vi "CreateWO-CompileDatatoSend.vi"(7 "Work Order":string, 8 "error in":errorcluster, 11 "ERP-CreateWorkOrder in":refnum<class "ERP-CreateWorkOrder.lvclass">) -> (0 "error out":errorcluster, 2 "Output JSON to DB":string, 3 "ERP-CreateWorkOrder out":refnum<class "ERP-CreateWorkOrder.lvclass">)   [LabVIEW 2013, in "ERP-CreateWorkOrder.lvclass"]
uses:
  ERP-CreateWorkOrder.lvclass
  ERP-CreateWorkOrder.lvclass/ERP-CreateWorkOrder.ctl
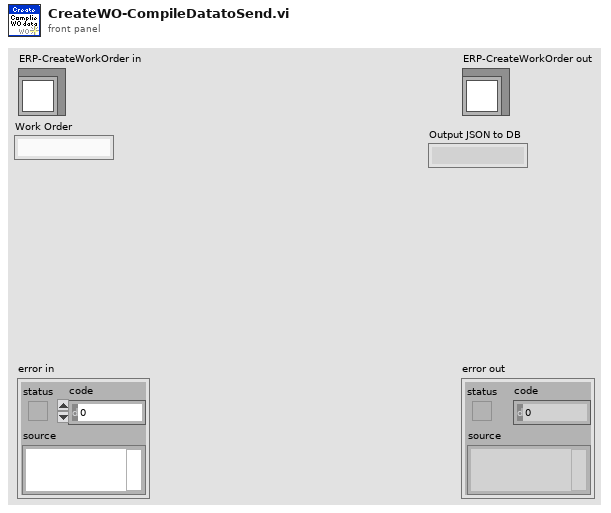
[diagram p1: front panel]
types:
  T1 = cluster{"Work Order":string, "Customer*":string, "Converted Start Date (String)":string, "Converted Due Date (String)":string, "Type Part Number*":string, "Part Number Description":string, "Quantity To Make":string, "Note - Special Instructions":string, "Assigned?":string, "Date Created":string, "Sales Order*":string, "Date Closed":string, "Status of Work Order":string, "Manufactured":string, "Inspected":string, "Approved":string, "Total Time to Manufacture":string, "Total Time to Inspect":string, "Path For PDF Special Instructions":string, "Reason For Closure":string, "RMA":string, "Manufacture User Notes":string, "Inspector User Notes":string, "Pull Inventory Note":string, "Stock Inventory Note":string}
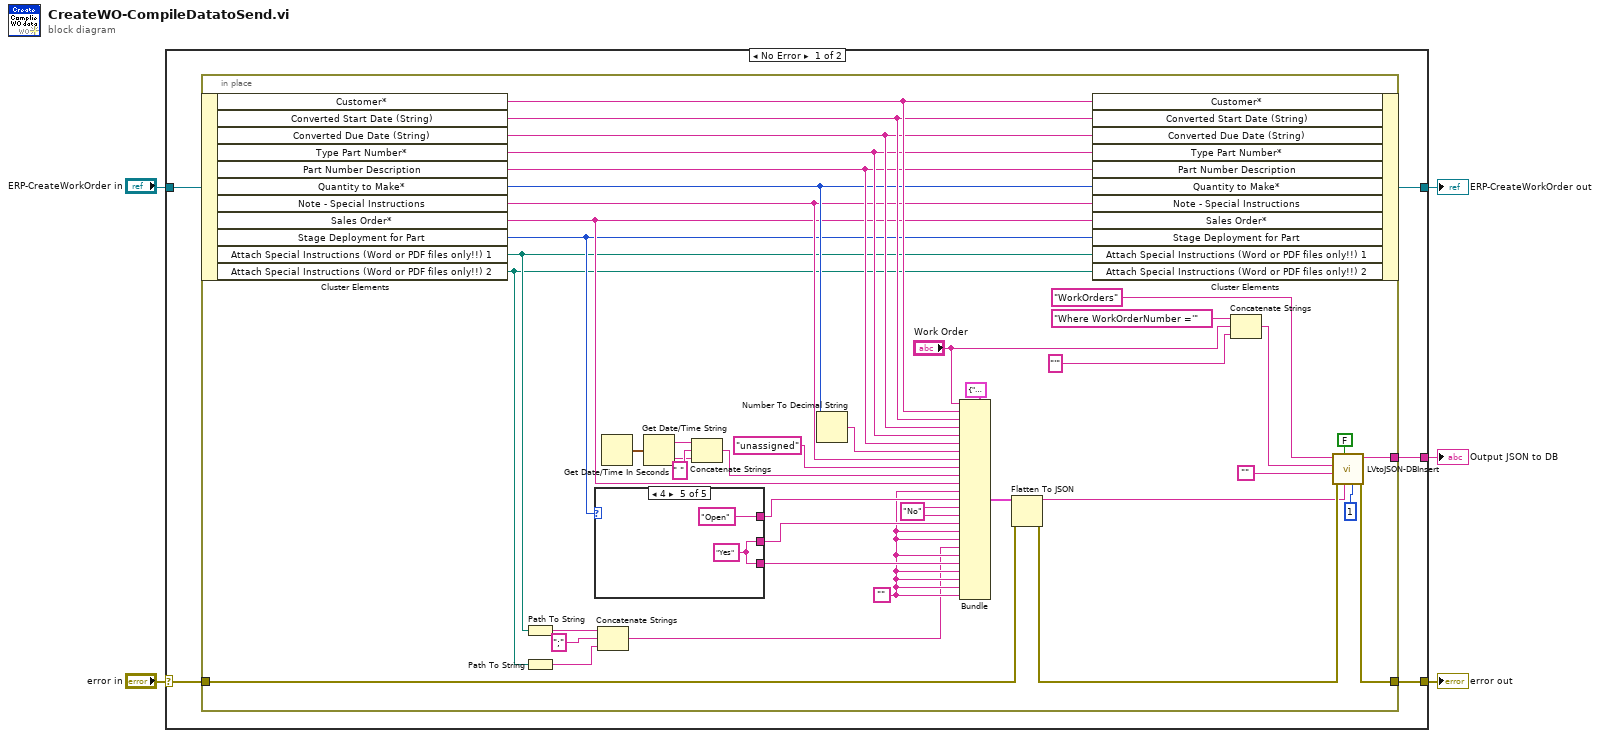
[diagram p0: block diagram]
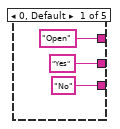
[diagram p2: hidden frame]
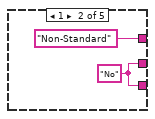
[diagram p3: hidden frame]
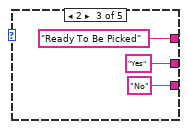
[diagram p4: hidden frame]
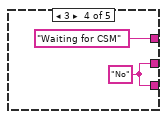
[diagram p5: hidden frame]
diagram:
  n1 = case shown="No Error" "error in" {
    selector: "error in" -> [w8 w66]
    tunnel: [w7 w66] -> w4
    tunnel: [w9 w65] -> w2
    tunnel: "ERP-CreateWorkOrder in" -> [w10 w65]
    tunnel: [w6 _] -> w1
    frame No Error {
      n2 = in-place {
        in-place-border: w8 -> [w17]
        in-place-border: [w30] -> w7
        in-place-border: [w29] -> w6
        w44 = "No" ("string")
        w25 = ""
        n3 = in-place-cluster #1(w10) -> ("Customer*"=w41:string, "Converted Start Date (String)"=w40:string, "Converted Due Date (String)"=w39:string, "Type Part Number*"=w38:string, "Part Number Description"=w37:string, "Quantity to Make*"=w36:i32, "Note - Special Instructions"=w35:string, "Sales Order*"=w34:string, "Stage Deployment for Part"=w33:u16, "Attach Special Instructions (Word or PDF files only!!) 1"=w24:path, "Attach Special Instructions (Word or PDF files only!!) 2"=w23:path)
        n4 = Path To String(path=w24) -> (string=w22:string)
        n5 = Path To String(path=w23) -> (string=w20:string)
        n6 = case shown="4" w33 {
          tunnel: ["Open" ("Status of Work Order") "Non-Standard" ("Status of Work Order") "Ready To Be Picked" ("Status of Work Order") "Waiting for CSM" ("Status of Work Order") "Open" ("Status of Work Order")] -> w45
          tunnel: ["Yes" ("Assigned?") w56 "Yes" ("Assigned?") w61 w63] -> w43
          tunnel: ["No" ("Assigned?") w56 "No" ("Assigned?") w61 w63] -> w42
          frame 0, Default {
          }
          frame 1 {
            w56 = "No" ("Assigned?")
          }
          frame 2 {
          }
          frame 3 {
            w61 = "No" ("Assigned?")
          }
          frame 4 {
            w63 = "Yes" ("Assigned?")
          }
        }
        n7 = Concatenate Strings(w22, ";" ("string"), w20) -> (w19:string)
        n8 = Get Date/Time In Seconds() -> (seconds since 1Jan1904=w50:timestamp)
        n9 = Get Date/Time String(seconds (now)=w50) -> (date string=w49:string, time string=w47:string)  [unwired: 2 in]
        n10 = Concatenate Strings(w49, " " ("string"), w47) -> (w46:string)
        n11 = Number To Decimal String(number=w36) -> (decimal integer string=w52:string)  [unwired: 1 in]
        n12 = Bundle(cluster=T1 {"Work Order"="", "Customer*"="", "Converted Start Date (String)"="", "Converted Due Date (String)"="", "Type Part Number*"="", "Part Number Description"="", "Quantity To Make"="", "Note - Special Instructions"="", "Assigned?"="", "Date Created"="", "Sales Order*"="", "Date Closed"="", "Status of Work Order"="", "Manufactured"="", "Inspected"="", "Approved"="", "Total Time to Manufacture"="", "Total Time to Inspect"="", "Path For PDF Special Instructions"="", "Reason For Closure"="", "RMA"="", "Manufacture User Notes"="", "Inspector User Notes"="", "Pull Inventory Note"="", "Stock Inventory Note"=""}, "Work Order"="Work Order", "Customer*"=w41, "Converted Start Date (String)"=w40, "Converted Due Date (String)"=w39, "Type Part Number*"=w38, "Part Number Description"=w37, "Quantity To Make"=w52, "Note - Special Instructions"=w35, "Assigned?"="unassigned", "Date Created"=w46, "Sales Order*"=w34, "Date Closed"=w25, "Status of Work Order"=w45, "Manufactured"=w44, "Inspected"=w44, "Approved"=w43, "Total Time to Manufacture"=w25, "Total Time to Inspect"=w25, "Path For PDF Special Instructions"=w19, "Reason For Closure"=w25, "RMA"=w42, "Manufacture User Notes"=w25, "Inspector User Notes"=w25, "Pull Inventory Note"=w25, "Stock Inventory Note"=w25) -> (w18:T1)
        n13 = Flatten To JSON(anything=w18, error in (no error)=w17) -> (JSON string=w15:string, 11:w16:errorcluster)  [unwired: 1 in]
        n14 = in-place-cluster #1("Customer*"=w41, "Converted Start Date (String)"=w40, "Converted Due Date (String)"=w39, "Type Part Number*"=w38, "Part Number Description"=w37, "Quantity to Make*"=w36, "Note - Special Instructions"=w35, "Sales Order*"=w34, "Stage Deployment for Part"=w33, "Attach Special Instructions (Word or PDF files only!!) 1"=w24, "Attach Special Instructions (Word or PDF files only!!) 2"=w23) -> (w9:refnum<class "ERP-CreateWorkOrder.lvclass">)
        n15 = Concatenate Strings("Where WorkOrderNumber ='" ("SQL Statement"), "Work Order", "'" ("string")) -> (w11:string)
        n16 = call "LVtoJSON-DBInsert.vi"("Type Of Insertion"=1, "Payload"=w15, "Update All"=FALSE, "error in"=w16, "Reply Command"="", "SQL Statement"=w11, "Table"="WorkOrders") -> ("error out"=w30:errorcluster, "Output JSON Object"=w29:string)  [unwired: 3 in]
      }
    }
    frame Error {
    }
  }
  "error out" <- w4
  "ERP-CreateWorkOrder out" <- w2
  "Output JSON to DB" <- w1
